vi "_ROSDefinition.vi"() -> ()   [LabVIEW 2010]
panel:
  in  "Queue Size":i32=10
  in  "TCP wait":i32=1000
  in  "Notifier Wait":i32=5000
  out "Ports":u16[](array[numeric])
  in  "FIFO Size":i32=10
  in  "Nodes":cluster{"node":string, "Node Port":i32}[](array[cluster])=[{"node"="/chris", "Node Port"=7000}]
  out "Robot There?":bool=TRUE
  out "ROS Master":string="192.168.1.110:11311"
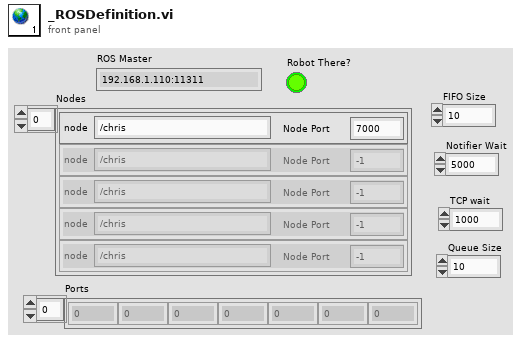
[diagram p1: front panel]
diagram:
